vi "update XorYwaveform.vi"(0 "AOparams":T1) -> (1 "outputwave":waveform(dbl), 2 "size":i32)   [LabVIEW 2015]
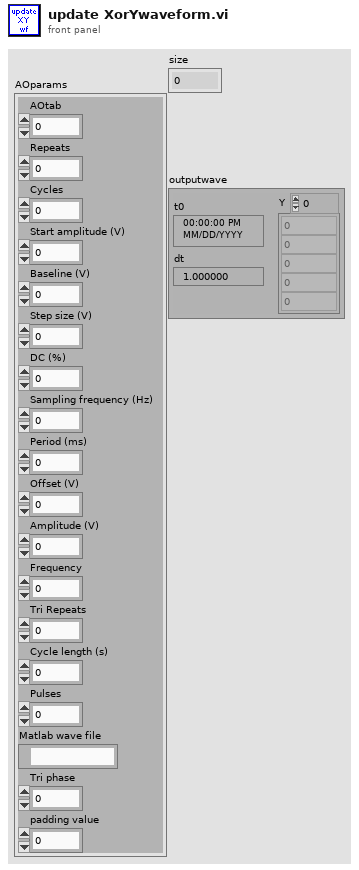
[diagram p1: front panel]
types:
  T1 = cluster{"AOtab":dbl, "Repeats":dbl, "Cycles":dbl, "Start amplitude (V)":dbl, "Baseline (V)":dbl, "Step size (V)":dbl, "DC (%)":dbl, "Sampling frequency (Hz)":dbl, "Period (ms)":dbl, "Offset (V)":dbl, "Amplitude (V)":dbl, "Frequency":dbl, "Tri Repeats":dbl, "Cycle length (s)":dbl, "Pulses":dbl, "Matlab wave file":path, "Tri phase":dbl, "padding value":dbl}
  T2 = typedef "LVRectTypeDef.ctl" = cluster{"Left":i16, "Top":i16, "Right":i16, "Bottom":i16}
  T3 = cluster{"Xpixels":i32, "Vxminref":dbl, "Vxmaxref":dbl, "P":dbl, "Ypixels":i32, "Vyminref":dbl, "Vymaxref":dbl, "srate":sgl, "sAOxy":i32, "timeout":dbl, "type":string, "date":string, "time":string, "Colormap":u16, "Drawing Mode":u16, "Scanning Mode":u16, "square pixels":bool, "square matrix":bool, "Xpixels Img":i32, "Vx-min Img":dbl, "VX-max Img":dbl, "Ypixels Img":i32, "Vy-min Img":dbl, "Vy-max Img ":dbl, "Angle Img":dbl, "autoshutter":bool, "finite":bool, "cont":bool, "wavdet":bool, "measpoints":i32, "avpp":i32, "bufferAO":i32, "bufferAI":i32, "starttick":u32, "waveform":path, "Vx-ref":dbl, "Vy-ref":dbl, "refreshrate":dbl, "refreshbuffer":i32, "tt_cycles":i32, "motorref":refnum<k7>, "mirrorswitch":refnum<k7>, "sample mode":i32, "maxbufferAI":i32, "srateAODO":sgl, "bin":sgl, "Pel":sgl, "Angle draw":dbl, "srate Img":sgl, "ROIimg_plotbounds":T2, "auto OD":bool, "ODfilt":u16, "aAI":i32[], "aCI":i32[], "aAO":u32[], "aDO":u32[], "refwfsize":dbl, "Lifetime":bool, "Vz-Img":dbl, "Vz-ref":dbl, "Vz-reset":dbl, "AIoverride":bool, "aAS":u32[], "XYZstart":dbl[], "External 100KHz Clock?":bool}
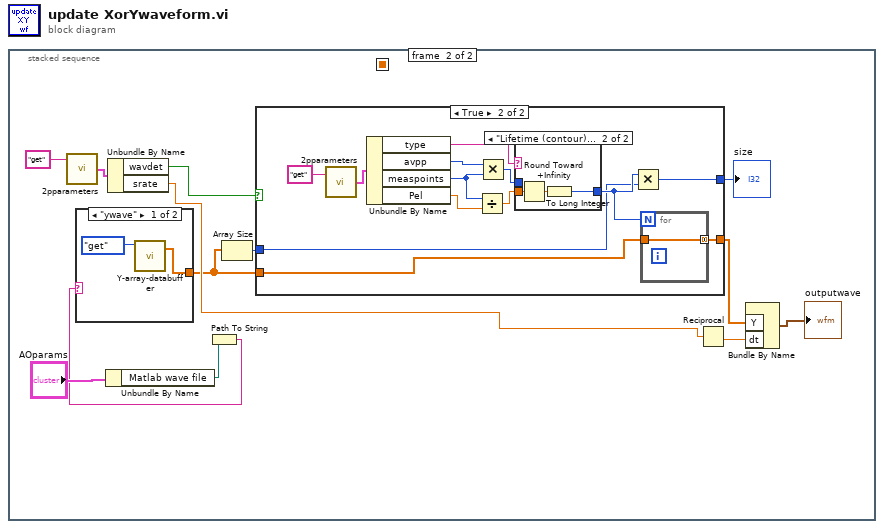
[diagram p0: block diagram]
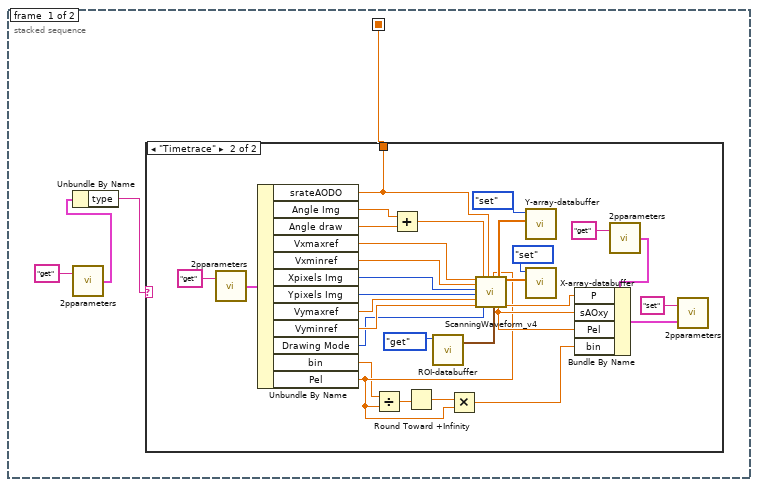
[diagram p2: hidden frame]
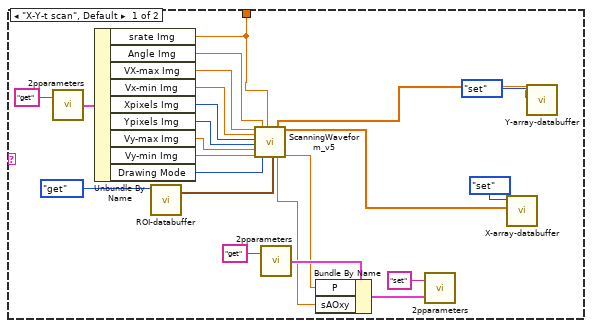
[diagram p3: hidden frame]
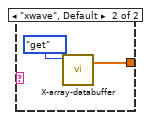
[diagram p6: hidden frame]
diagram:
  n1 = stacked-sequence {
    seq-local: [w4 _] -> [_ _]
    frame #0 {
      n2 = call "2pparameters.vi"("command"="get") -> ("params out"=w2:T3)  [unwired: 1 in]
      n3 = Unbundle By Name(w2) -> ("type"=w1:string)
      n4 = case shown="\"Timetrace\"" w1 {
        tunnel: [w5 w28] -> w4
        frame "X-Y-t scan", Default {
          n5 = call "2pparameters.vi"("command"="get") -> ("params out"=w19:T3)  [unwired: 1 in]
          n6 = Unbundle By Name(w19) -> ("srate Img"=w5:sgl, "Angle Img"=w18:dbl, "VX-max Img"=w17:dbl, "Vx-min Img"=w16:dbl, "Xpixels Img"=w15:i32, "Ypixels Img"=w14:i32, "Vy-max Img"=w13:dbl, "Vy-min Img"=w12:dbl, "Drawing Mode"=w11:u16)
          n7 = call "ROI-databuffer.vi"("command"=enum16{"get", "set", "clear", "append"}."get") -> ("array out"=w10:cluster{"x":sgl, "y":sgl}[])  [unwired: 4 in]
          n8 = call "ScanningWaveform_v5.vi"("Vy-min"=w12, "Vy-max"=w13, "yPixels/tPixels"=w14, "xPixels/rPixels"=w15, "Vx-min"=w16, "Vx-max"=w17, "Drawing Mode"=w11, "Angle"=w18, "AOrate"=w5, "Points"=w10) -> ("numPixels"=w6:dbl, "Y-WaveArray"=w9:dbl[], "P"=w7:dbl, "X-WaveArray"=w8:dbl[])  [unwired: 6 in]
          n9 = call "2pparameters.vi"("command"="get") -> ("params out"=w27:T3)  [unwired: 1 in]
          n10 = Bundle By Name(cluster=w27, "P"=w7, "sAOxy"=w6) -> (w24:T3)
          n11 = call "2pparameters.vi"("Params in"=w24, "command"="set") -> ()  [unwired: 1 out]
          n12 = call "X-array-databuffer.vi"("array in"=w8, "command"=enum16{"get", "set", "clear", "append"}."set") -> ()  [unwired: 2 in, 2 out]
          n13 = call "Y-array-databuffer.vi"("array in"=w9, "command"=enum16{"get", "set", "clear", "append"}."set") -> ()  [unwired: 2 in, 2 out]
        }
        frame "Timetrace" {
          n14 = call "2pparameters.vi"("command"="get") -> ("params out"=w41:T3)  [unwired: 1 in]
          n15 = Unbundle By Name(w41) -> ("srateAODO"=w28:sgl, "Angle Img"=w40:dbl, "Angle draw"=w39:dbl, "Vxmaxref"=w38:dbl, "Vxminref"=w37:dbl, "Xpixels Img"=w36:i32, "Ypixels Img"=w35:i32, "Vymaxref"=w34:dbl, "Vyminref"=w33:dbl, "Drawing Mode"=w32:u16, "bin"=w29:sgl, "Pel"=w30:sgl)
          n16 = Divide(x=w29, y=w30) -> (x/y=w55:sgl)
          n17 = Add(x=w40, y=w39) -> (x+y=w57:dbl)
          n18 = Round Toward +Infinity(x=w55) -> (ceil(x): smallest int >= x=w56:sgl)
          n19 = call "ROI-databuffer.vi"("command"=enum16{"get", "set", "clear", "append"}."get") -> ("array out"=w47:cluster{"x":sgl, "y":sgl}[])  [unwired: 4 in]
          n20 = Multiply(x=w56, y=w30) -> (x*y=w31:sgl)
          n21 = call "ScanningWaveform_v4.vi"("Vy-min"=w33, "Vy-max"=w34, "yPixels/tPixels"=w35, "xPixels/rPixels"=w36, "Vx-min"=w37, "Vx-max"=w38, "Drawing Mode"=w32, "Angle"=w57, "AOrate"=w28, "Points"=w47, "points in ellipse"=w30) -> ("numPixels"=w54:dbl, "Y-WaveArray"=w53:dbl[], "P"=w48:dbl, "X-WaveArray"=w52:dbl[])  [unwired: 5 in]
          n22 = call "Y-array-databuffer.vi"("array in"=w53, "command"=enum16{"get", "set", "clear", "append"}."set") -> ()  [unwired: 2 in, 2 out]
          n23 = call "X-array-databuffer.vi"("array in"=w52, "command"=enum16{"get", "set", "clear", "append"}."set") -> ()  [unwired: 2 in, 2 out]
          n24 = call "2pparameters.vi"("command"="get") -> ("params out"=w43:T3)  [unwired: 1 in]
          n25 = Bundle By Name(cluster=w43, "P"=w48, "sAOxy"=w54, "Pel"=w54, "bin"=w31) -> (w51:T3)
          n26 = call "2pparameters.vi"("Params in"=w51, "command"="set") -> ()  [unwired: 1 out]
        }
      }
    }
    frame #1 {
      n27 = call "2pparameters.vi"("command"="get") -> ("params out"=w63:T3)  [unwired: 1 in]
      n28 = Unbundle By Name("AOparams") -> ("Matlab wave file"=w69:path)
      n29 = Unbundle By Name(w63) -> ("wavdet"=w62:bool, "srate"=w61:sgl)
      n30 = Path To String(path=w69) -> (string=w68:string)
      n31 = case shown="\"ywave\"" w68 {
        tunnel: [w91 w93] -> w60
        frame "ywave" {
          n32 = call "Y-array-databuffer.vi"("command"=enum16{"get", "set", "clear", "append"}."get") -> ("array out"=w91:dbl[])  [unwired: 3 in, 1 out]
        }
        frame "xwave", Default {
          n33 = call "X-array-databuffer.vi"("command"=enum16{"get", "set", "clear", "append"}."get") -> ("array out"=w93:dbl[])  [unwired: 3 in, 1 out]
        }
      }
      n34 = Array Size(array=w60) -> (size(s)=w59:i32)
      n35 = case shown="True" w62 {
        tunnel: w60 -> [w72 w77]
        tunnel: [w72 w76] -> w65
        tunnel: w59 -> [w71 w74]
        tunnel: [w71 w73] -> w58
        frame False {
        }
        frame True {
          n36 = call "2pparameters.vi"("command"="get") -> ("params out"=w80:T3)  [unwired: 1 in]
          n37 = Unbundle By Name(w80) -> ("type"=w83:string, "avpp"=w78:i32, "measpoints"=w81:i32, "Pel"=w82:sgl)
          n38 = Divide(x=w81, y=w82) -> (x/y=w84:sgl)
          n39 = Multiply(x=w78, y=w81) -> (x*y=w85:i32)
          n40 = case shown="\"Lifetime (contour)\", \"Timetrace\"" w83 {
            tunnel: w84 -> [_ w89]
            tunnel: [w86 w87] -> w75
            tunnel: w85 -> [w86 _]
            frame "Lifetime (scan)", "X-Y-Z stack", "X-Y-t movie", Default {
            }
            frame "Lifetime (contour)", "Timetrace" {
              n41 = Round Toward +Infinity(x=w89) -> (ceil(x): smallest int >= x=w88:sgl)
              n42 = To Long Integer(number=w88) -> (32bit integer=w87:i32)
            }
          }
          n43 = Multiply(x=w75, y=w74) -> (x*y=w73:i32)
          n44 = for {
            N: w75 -> [_]
            tunnel: w77 -> [w90]
            tunnel: [w90] -> w76 mode=concatenating
          }
        }
      }
      "size" <- w58
      n45 = Reciprocal(x=w61) -> (1/x=w67:sgl)
      n46 = Bundle By Name("Y"=w65, "dt"=w67) -> (→"outputwave":waveform(dbl))  [unwired: 1 in]
    }
  }
